vi "thermo_check_retry.vi"(8 "error in":errorcluster, 9 "thermo error in":errorcluster, 11 "thermo in":T1={"type"=enum."COMET Tx5xx (ethernet)", "comment"="", "tag"="", "refresh"=5.0, "IP"="192.168.2.34", "port"=502, "VISA"="", "last readout"=timestamp(0 s since 1904-01-01), "TCP ref"=refnum, "VISA sess"="", "idn"="", "press"=0.0, "RH"=0.0, "temp"=0.0, "pres cor"=[], "RH cor"=[], "temp cor"=[], "try left"=0, "failed"=FALSE, "RTD set"=[], "RTD inv"=[], "range"=0.0, "net mode"=enum."MODBUS", "try fail"=enum."Stop trying - return NaN", "timeout [s]"=0.0, "max retries"=0, "sim t [deg]"=0.0} {"RTD inv" format="%.1f"; "RTD set" format="%.1f"; "temp cor" format="%.1f"; "RH cor" format="%.1f"; "pres cor" format="%.1f"; "refresh" min=0.1 max=1000.0 format="%.2f"}) -> (0 "error out":errorcluster, 1 "fail":bool, 2 "retry":bool, 3 "thermo out":T1={"type"=enum."COMET Tx5xx (ethernet)", "comment"="", "tag"="", "refresh"=5.0, "IP"="192.168.2.34", "port"=502, "VISA"="", "last readout"=timestamp(0 s since 1904-01-01), "TCP ref"=refnum, "VISA sess"="", "idn"="", "press"=0.0, "RH"=0.0, "temp"=0.0, "pres cor"=[], "RH cor"=[], "temp cor"=[], "try left"=0, "failed"=FALSE, "RTD set"=[], "RTD inv"=[], "range"=0.0, "net mode"=enum."MODBUS", "try fail"=enum."Stop trying - return NaN", "timeout [s]"=0.0, "max retries"=0, "sim t [deg]"=0.0} {"RTD inv" format="%.1f"; "RTD set" format="%.1f"; "temp cor" format="%.1f"; "RH cor" format="%.1f"; "pres cor" format="%.1f"; "refresh" min=0.1 max=1000.0 format="%.2f"})   [LabVIEW 2020]
uses:
  thermo.ctl
  thermo_types.ctl
  Thermometer Fail Action.ctl
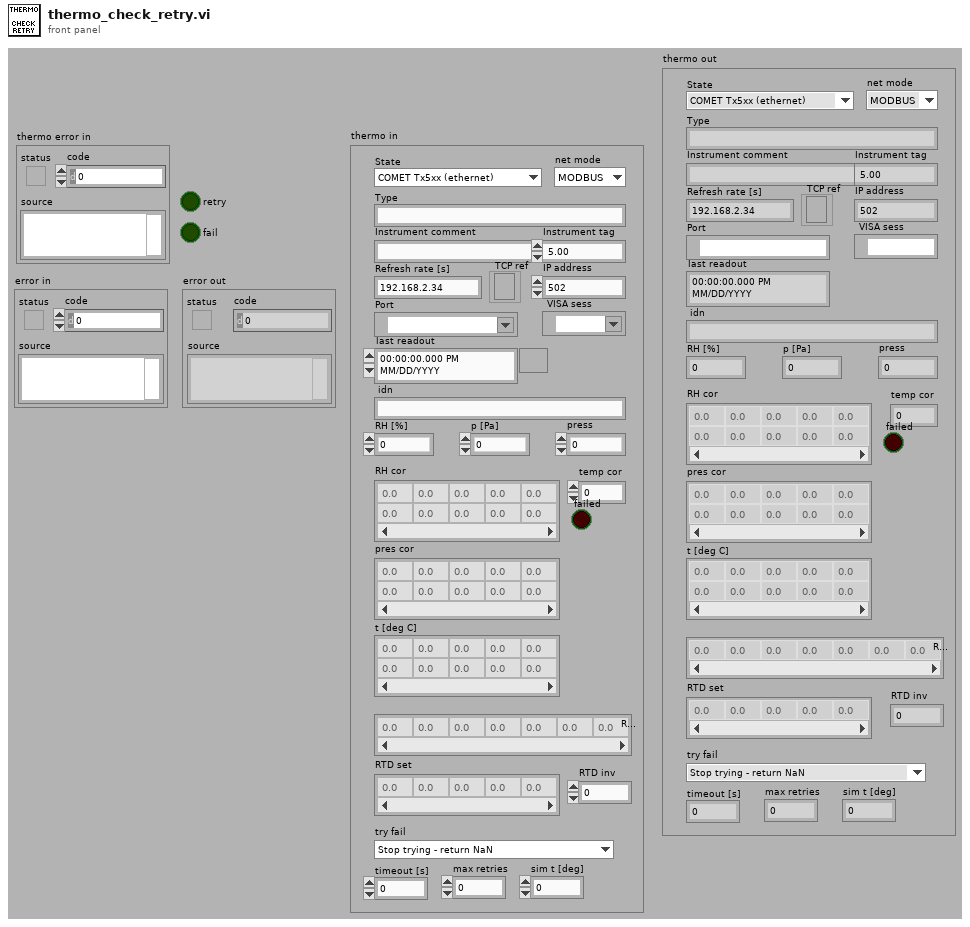
[diagram p1: front panel]
types:
  T1 = typedef "thermo.ctl" = cluster{"type":T2, "comment":string, "tag":string, "refresh":dbl, "IP":string, "port":u16, "VISA":refnum<visa-resource-name>, "last readout":timestamp, "TCP ref":refnum<k5>, "VISA sess":refnum<visa-resource-name>, "idn":string, "press":dbl, "RH":dbl, "temp":dbl, "pres cor":dbl[][], "RH cor":dbl[][], "temp cor":dbl[][], "try left":i32, "failed":bool, "RTD set":dbl[], "RTD inv":dbl[], "range":dbl, "net mode":enum16{"MODBUS", "HTTP"}, "try fail":T3, "timeout [s]":dbl, "max retries":i32, "sim t [deg]":dbl}
  T2 = typedef "thermo_types.ctl" = enum16{"Disabled", "Simulated", "COMET Tx5xx (ethernet)", "Keithley 2002 (GPIB) + RTD", "Agilent 344xx (GPIB) + RTD"}
  T3 = typedef "Thermometer Fail Action.ctl" = enum16{"Stop trying - keep last value", "Stop trying - return NaN", "Generate error - stop sweep"}
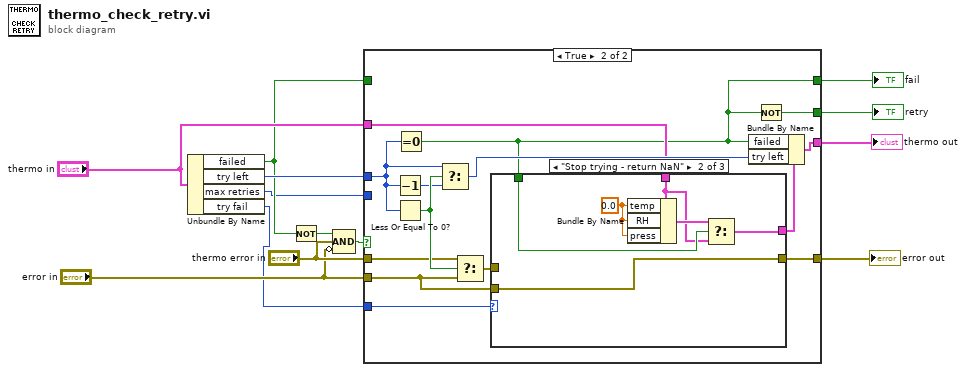
[diagram p0: block diagram]
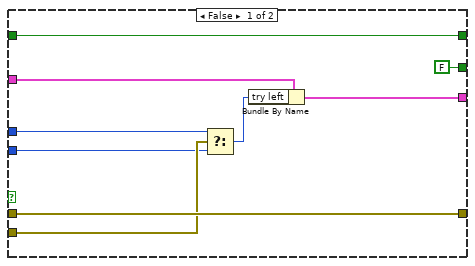
[diagram p2: hidden frame]
diagram:
  n1 = Unbundle By Name("thermo in") -> ("failed"=w3:bool, "try left"=w12:i32, "max retries"=w2:i32, "try fail"=w1:T3)
  n2 = Not(x=w3) -> (.not. x?=w7:bool)
  n3 = Compound Arithmetic op=AND(w7, "thermo error in", invert "error in") -> (w8:bool)
  n4 = case shown="True" w8 {
    tunnel: [w20 w36] -> w13
    tunnel: w12 -> [w18 w27]
    tunnel: "error in" -> [w19 w29]
    tunnel: "thermo in" -> [w22 w31]
    tunnel: [w21 w34] -> w11
    tunnel: [FALSE w26] -> w9
    tunnel: "thermo error in" -> [w20 w25]
    tunnel: [w16 w24] -> w4
    tunnel: w3 -> [w16 _]
    tunnel: w2 -> [w14 _]
    tunnel: w1 -> [_ w23]
    frame False {
      n5 = Select(t=w18, s=w19, f=w14) -> (s? t:f=w17:i32)
      n6 = Bundle By Name(cluster=w22, "try left"=w17) -> (w21:T1)
    }
    frame True {
      n7 = Decrement(x=w27) -> (x-1=w28:i32)
      n8 = Less Or Equal To 0?(x=w27) -> (x <= 0?=w33:bool)
      n9 = Equal To 0?(x=w27) -> (x = 0?=w24:bool)
      n10 = Select(t=w27, s=w33, f=w28) -> (s? t:f=w32:i32)
      n11 = Select(t=w25, s=w33, f=w29) -> (s? t:f=w35:errorcluster)
      n12 = case shown="\"Stop trying - return NaN\"" w23 {
        tunnel: w29 -> [w38 w43 _]
        tunnel: [w38 w43 w46] -> w36
        tunnel: w35 -> [_ _ w46]
        tunnel: w24 -> [_ w41 _]
        tunnel: w31 -> [w37 w39 w45]
        tunnel: [w37 w42 w45] -> w30
        frame "Stop trying - keep last value", Default {
        }
        frame "Stop trying - return NaN" {
          w44 = 0.0 ("temp")
          n13 = Bundle By Name(cluster=w39, "temp"=w44, "RH"=w44, "press"=w44) -> (w40:T1)
          n14 = Select(t=w40, s=w41, f=w39) -> (s? t:f=w42:T1)
        }
        frame "Generate error - stop sweep" {
        }
      }
      n15 = Bundle By Name(cluster=w30, "failed"=w24, "try left"=w32) -> (w34:T1)
      n16 = Not(x=w24) -> (.not. x?=w26:bool)
    }
  }
  "error out" <- w13
  "thermo out" <- w11
  "retry" <- w9
  "fail" <- w4
